vi "Engine-RPC-SyncPumpA.vi"(8 "Error In":errorcluster, 11 "DSI Reference":refnum<class "DCM-DSI.lvclass">) -> (0 "Error Out":errorcluster, 3 "DSI Reference":refnum<class "DCM-DSI.lvclass">)   [LabVIEW 2016, in "DSI-RT.lvlib"]
uses:
  DSI-RT.lvlib
  Classes/DCM-DSI/DCM-DSI.lvclass
  <vilib>/addons/Software Calibration Management/xSCM/Controls/TBL2D.ctl
  <vilib>/Powertrain Controls/Device Drivers/DCM/Rev0/RT/DCM - RT.lvclass/DCM - RT.ctl
  <vilib>/Powertrain Controls/Device Drivers/DCM/Rev0/RT/Read Max CAD.vi
  Classes/DCM-DSI/Read DiffIO Results.vi
  Classes/DCM-DSI/Read DCM Ref.vi
  Classes/DCM-DSI/Read EPTx Data.vi
  Classes/DCM-DSI/Read Channels.vi
  Classes/DCM-DSI/Read dt.vi
  Classes/DCM-DSI/Write Pump-A Command.vi
  <vilib>/Powertrain Controls/Device Drivers/DCM/Rev0/RT/DCM - RT.lvclass
  <vilib>/addons/Software Calibration Management/xSCM/FaultPoint.xnode
  <vilib>/addons/Software Calibration Management/xSCM/CalPoint.xnode
  <vilib>/addons/Software Calibration Management/xSCM/Controls/TLU2D.ctl
  <vilib>/addons/Software Calibration Management/xSCM/ni_scm.dll
  <vilib>/addons/Software Calibration Management/xSCM/SCM-API.lvlib
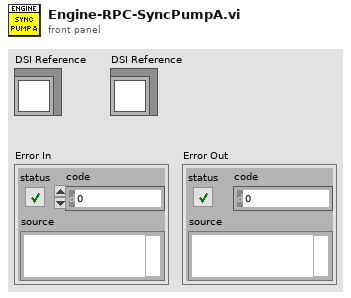
[diagram p1: front panel]
types:
  T1 = cluster{"PID_Kp":sgl, "PID_Ti":sgl, "PID_Td":sgl, "PID_FF":sgl, "Non-PID_FF":sgl, "PID_Min":sgl, "PID_Max":sgl}
  T2 = typedef "DCM - RT - Diff IO.lvlib/Results.ctl" = cluster{"Capture [DBTDC]":sgl, "Capture Error":bool, "Frequency [Hz]":sgl, "Duty Cycle [%]":sgl, "PWM Stopped":bool}
  T3 = typedef "EPTx - RevA - RT.lvlib/EPTxData.ctl" = cluster{"Sync":bool, "CurrentCAD":sgl, "Speed [RPM]":sgl, "Config":bool, "Rcvg Primary":bool, "Stall":bool, "Overflow":bool, "Ratio Error":bool, "Pattern Error":bool, "Aux Warning":bool, "Watchdog Error":bool}
  T4 = typedef "DCM-DSI.lvclass/Channel.ctl" = cluster{"Name":string, "Unit":string, "Value":sgl}
  T5 = typedef "DSI-Shared.lvlib/Engine-Channel.ctl" = cluster{"Name":string, "Unit":string, "Value":sgl}
  T6 = typedef "SCM-API.lvlib/TBL2D.ctl" = cluster{"X":sgl[], "Y":sgl[], "Z":sgl[][]}
  T7 = typedef "SCM-API.lvlib/TLU2D.ctl" = cluster{"X":sgl, "Y":sgl, "Z":sgl}
  T8 = cluster{"Duration":cluster{"Dur_Max":sgl, "Dur_Min":sgl, "Dur_ManE":bool, "Dur_Man":sgl}, "Timing":cluster{"WindowStart":sgl, "WindowEnd":sgl, "EndAngle?":bool, "DurAngle_Max":sgl, "MinOffTime":sgl}}
  T9 = cluster{"Dur_Max":sgl, "Dur_Min":sgl, "Dur_ManE":bool, "Dur_Man":sgl}
  T10 = cluster{"WindowStart":sgl, "WindowEnd":sgl, "EndAngle?":bool, "DurAngle_Max":sgl, "MinOffTime":sgl}
  T11 = cluster{"ProportionalAction":sgl, "IntegralAction":sgl, "DerivativeAction":sgl}
  T12 = enum8{"Unused", "User OS", "Diff IO 1", "Diff IO 2", "Diff IO 3", "Diff IO 4", "Diff IO 5", "Diff IO 6", "Diff IO 7", "Diff IO 8", "Aux 1", "Aux 2", "Aux 3", "Aux 4", "Aux 5", "Aux 6", "Aux 7", "Aux 8", "Aux 9", "Aux 10", "Aux 11", "Aux 12", "Aux 13", "Aux 14", "Aux 15", "Aux 16"}
  T13 = cluster{"Value":enum8{"Unused", "User OS", "Diff IO 1", "Diff IO 2", "Diff IO 3", "Diff IO 4", "Diff IO 5", "Diff IO 6", "Diff IO 7", "Diff IO 8", "Aux 1", "Aux 2", "Aux 3", "Aux 4", "Aux 5", "Aux 6", "Aux 7", "Aux 8", "Aux 9", "Aux 10", "Aux 11", "Aux 12", "Aux 13", "Aux 14", "Aux 15", "Aux 16"}, "Value":sgl}
  T14 = cluster{"Value":sgl, "Value":sgl, "Duration_Output":sgl}
  T15 = typedef "DCM - RT - DI.lvlib/Command.ctl" = cluster{"Mode":T16, "Digital Input":T17, "Default Profile Index":u8, "Cal Freq [Hz]":sgl, "Cal Duration [s]":sgl, "Cal Increment [s]":sgl, "Cal Pulses":u16, "TMP Command Sequence":T18[], "EPT TDC Offset [CAD]":sgl, "EPT Window Start [DBTDC]":sgl, "EPT Window End [DBTDC]":sgl, "EPT Angles":T19[], "EPT Skip Fire":bool, "EPT Skip Index":u8, "EPT Precharge Duration [s]":sgl, "EPT Precharge Profile Index":u8}
  T16 = typedef "DCM - FPGA - DI.lvlib/Mode.ctl" = enum8{"Off", "Direct", "Calibration", "Triggered Multi-Pulse", "Engine Position Tracking"}
  T17 = typedef "DCM - FPGA.lvlib/Digital Channel.ctl" = enum8{"Unused", "User OS", "Diff IO 1", "Diff IO 2", "Diff IO 3", "Diff IO 4", "Diff IO 5", "Diff IO 6", "Diff IO 7", "Diff IO 8", "Aux 1", "Aux 2", "Aux 3", "Aux 4", "Aux 5", "Aux 6", "Aux 7", "Aux 8", "Aux 9", "Aux 10", "Aux 11", "Aux 12", "Aux 13", "Aux 14", "Aux 15", "Aux 16"}
  T18 = typedef "DCM - RT - DI.lvlib/Command Sequence.ctl" = cluster{"Duration [s]":sgl, "Level":bool, "Run/Stop":bool, "Profile Index":u8}
  T19 = typedef "DCM - RT - DI.lvlib/Angle Control.ctl" = cluster{"Enable":bool, "Timing [DBTDC]":sgl, "Duration [s]":sgl, "Profile Index":u8}
  T20 = cluster{"Sync-A_Timing":sgl, "Sync-A_CamAdv":sgl}
  T21 = cluster{"Output":cluster{"Duration_Output":sgl, "PID_Output":sgl}, "EPT Mode Output":cluster{"Sync-A_Timing":sgl, "Sync-A_CamAdv":sgl}, "TMP Mode Output":cluster{"Sync-A_Delay":sgl, "Sync-A_Period":sgl}}
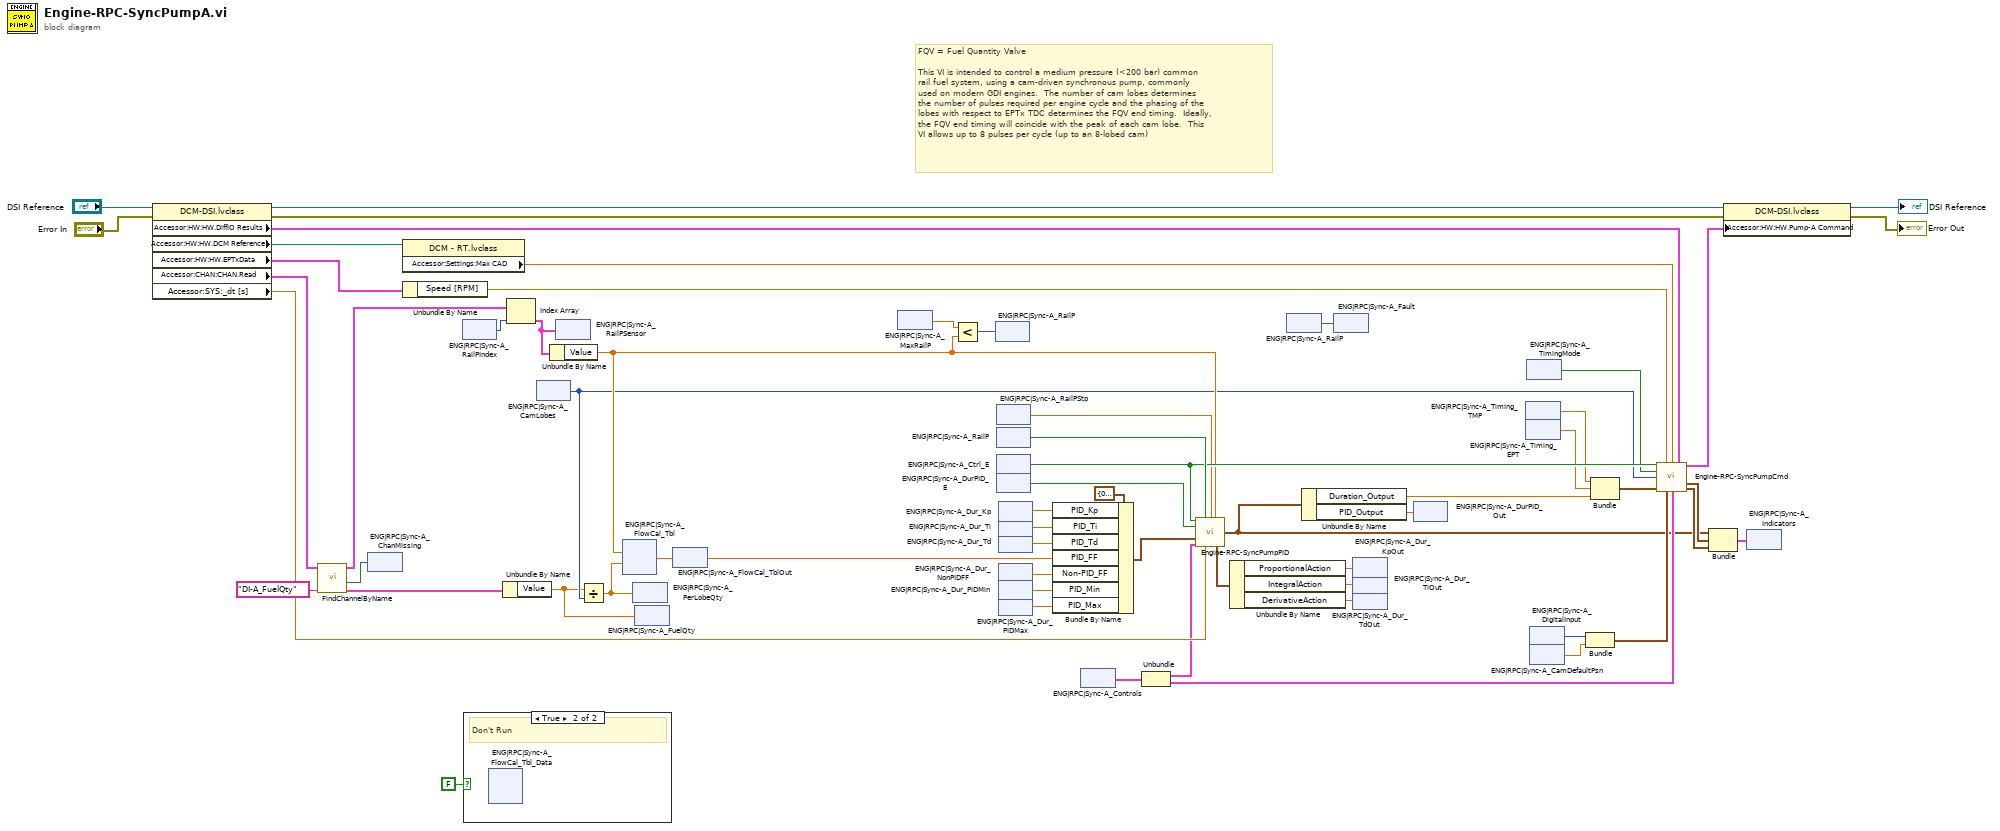
[diagram p0: block diagram]
diagram:
  # "FQV = Fuel Quantity Valve\n\nThis VI is intended to control a medium pressure (<200 bar) common\nrail fuel system, using a cam-driven synchronous pump, commonly\nused on modern GDI engines.  The number of cam lobes determines \nthe number of pulses required per engine cycle and the phasing of the\nlobes with respect to EPTx TDC determines the FQV end timing.  Ideally,\nthe FQV end timing will coincide with the peak of each cam lobe.  This\nVI allows up to 8 pulses per cycle (up to an 8-lobed cam)"
  n1 = property class="DCM-DSI.lvclass"(reference="DSI Reference", error in="Error In") -> (reference out=w44:refnum<class "DCM-DSI.lvclass">, error out=w43:errorcluster, "Accessor:HW:HW.DiffIO Results"=w30:T2[], "Accessor:HW:HW.DCM Reference"=w31:refnum<class "DCM - RT.lvclass">, "Accessor:HW:HW.EPTxData"=w42:T3, "Accessor:CHAN:CHAN.Read"=w7:T4[], "Accessor:SYS:_dt [s]"=w39:sgl)
  n2 = call "FindChannelByName.vi"("Name"="DI-A_FuelQty", "CTRL.Channels in"=w7) -> ("Channel"=w9:T5, "Searching"=w5:bool, "CTRL.Channels out"=w4:T5[])  [unwired: 6 in, 1 out]
  n3 = xnode "ENG|RPC|Sync-A_ChanMissing"("Fault"=w5) -> ()
  n4 = property class="DCM - RT.lvclass"(reference=w31) -> ("Accessor:Settings:Max CAD"=w32:sgl)  [unwired: 1 in, 2 out]
  n5 = Unbundle By Name(w42) -> ("Speed [RPM]"=w35:sgl)
  n6 = xnode "ENG|RPC|Sync-A_RailPIndex"() -> ("Value"=w3:i32)
  n7 = case shown="True" FALSE {
    frame False {
    }
    frame True {
      # "Don't Run"
      n8 = xnode "ENG|RPC|Sync-A_FlowCal_Tbl_Data"() -> ()  [unwired: 1 out]
    }
  }
  n9 = Unbundle By Name(w9) -> ("Value"=w10:sgl)
  n10 = Index Array(array=w4, index=w3) -> (element=w2:T5)
  n11 = xnode "ENG|RPC|Sync-A_CamLobes"() -> ("Value"=w20:u8)
  n12 = Unbundle By Name(w2) -> ("Value"=w21:sgl)
  n13 = xnode "ENG|RPC|Sync-A_RailPSensor"("Value"=w2) -> ()
  n14 = Divide(x=w10, y=w20) -> (x/y=w37:sgl)
  n15 = xnode "ENG|RPC|Sync-A_FlowCal_Tbl"("Y Index"=w37, "X Index"=w21) -> ("Z"=w45:sgl)
  n16 = xnode "ENG|RPC|Sync-A_PerLobeQty"("Value"=w37) -> ()
  n17 = xnode "ENG|RPC|Sync-A_FuelQty"("Value"=w10) -> ()
  n18 = xnode "ENG|RPC|Sync-A_FlowCal_TblOut"("Value"=w45) -> ()
  n19 = xnode "ENG|RPC|Sync-A_MaxRailP"() -> ("Value"=w22:sgl)
  n20 = Less?(x=w22, y=w21) -> (x < y?=w41:bool)
  n21 = xnode "ENG|RPC|Sync-A_RailP"("Fault"=w41) -> ()
  n22 = xnode "ENG|RPC|Sync-A_RailPStp"() -> ("Value"=w12:sgl)
  n23 = xnode "ENG|RPC|Sync-A_RailP"() -> ("Fault"=w40:bool)
  n24 = xnode "ENG|RPC|Sync-A_Ctrl_E"() -> ("Value"=w36:bool)
  n25 = xnode "ENG|RPC|Sync-A_DurPID_E"() -> ("Value"=w46:bool)
  n26 = xnode "ENG|RPC|Sync-A_Dur_Kp"() -> ("Value"=w50:sgl)
  n27 = xnode "ENG|RPC|Sync-A_Dur_Ti"() -> ("Value"=w51:sgl)
  n28 = xnode "ENG|RPC|Sync-A_Dur_Td"() -> ("Value"=w52:sgl)
  n29 = xnode "ENG|RPC|Sync-A_Dur_NonPIDFF"() -> ("Value"=w38:sgl)
  n30 = xnode "ENG|RPC|Sync-A_Dur_PIDMin"() -> ("Value"=w53:sgl)
  n31 = xnode "ENG|RPC|Sync-A_Dur_PIDMax"() -> ("Value"=w54:sgl)
  n32 = Bundle By Name(cluster=T1 {"PID_Kp"=0.0, "PID_Ti"=0.01, "PID_Td"=0.0, "PID_FF"=0.0, "Non-PID_FF"=0.0, "PID_Min"=-100.0, "PID_Max"=100.0} ("PID Settings"), "PID_Kp"=w50, "PID_Ti"=w51, "PID_Td"=w52, "PID_FF"=w45, "Non-PID_FF"=w38, "PID_Min"=w53, "PID_Max"=w54) -> (w47:T1)
  n33 = xnode "ENG|RPC|Sync-A_Controls"() -> ("Value"=w19:T8)
  n34 = Unbundle(w19) -> ("Duration"=w18:T9, "Timing"=w17:T10)
  n35 = call "Engine-RPC-SyncPumpPID.vi"("Control Enable"=w36, "Fault Input"=w40, "Rail Press Setpoint"=w12, "Rail Pressure"=w21, "PID Enable"=w46, "PID Settings"=w47, "Output Management Controls"=w18, "dt (s)"=w39) -> ("Output"=w14:cluster{"Duration_Output":sgl, "PID_Output":sgl}, "PID_Action_Output"=w49:T11)  [unwired: 6 in]
  n36 = Unbundle By Name(w49) -> ("ProportionalAction"=w57:sgl, "IntegralAction"=w56:sgl, "DerivativeAction"=w55:sgl)
  n37 = xnode "ENG|RPC|Sync-A_RailP"() -> ("Fault"=w6:bool)
  n38 = Unbundle By Name(w14) -> ("Duration_Output"=w24:sgl, "PID_Output"=w11:sgl)
  n39 = xnode "ENG|RPC|Sync-A_Fault"("Value"=w6) -> ()
  n40 = xnode "ENG|RPC|Sync-A_Dur_KpOut"("Value"=w57) -> ()
  n41 = xnode "ENG|RPC|Sync-A_Dur_TiOut"("Value"=w56) -> ()
  n42 = xnode "ENG|RPC|Sync-A_Dur_TdOut"("Value"=w55) -> ()
  n43 = xnode "ENG|RPC|Sync-A_DurPID_Out"("Value"=w11) -> ()
  n44 = xnode "ENG|RPC|Sync-A_Timing_TMP"() -> ("Value"=w26:sgl)
  n45 = xnode "ENG|RPC|Sync-A_Timing_EPT"() -> ("Value"=w25:sgl)
  n46 = xnode "ENG|RPC|Sync-A_TimingMode"() -> ("Value"=w27:bool)
  n47 = xnode "ENG|RPC|Sync-A_DigitalInput"() -> ("Value"=w34:T12)
  n48 = xnode "ENG|RPC|Sync-A_CamDefaultPsn"() -> ("Value"=w33:sgl)
  n49 = Bundle("Value"=w34, "Value"=w33) -> (w28:T13)  [unwired: 1 in]
  n50 = Bundle("Value"=w26, "Value"=w25, "Duration_Output"=w24) -> (w23:T14)  [unwired: 1 in]
  n51 = call "Engine-RPC-SyncPumpCmd.vi"("FQV Enable"=w36, "Engine Speed [RPM]"=w35, "MaxCAD"=w32, "HW.DiffIO Results"=w30, "Mode [T=Trig,F=EPT]"=w27, "Cam Lobes"=w20, "Command"=w23, "DigitalInputSettings"=w28, "EPT Mode Settings"=w17) -> ("Pump Command"=w29:T15, "EPT Mode Output"=w16:T20, "TMP Mode Output"=w15:cluster{"Sync-A_Delay":sgl, "Sync-A_Period":sgl})  [unwired: 4 in]
  n52 = Bundle("Output"=w14, "EPT Mode Output"=w16, "TMP Mode Output"=w15) -> (w13:T21)  [unwired: 1 in]
  n53 = property class="DCM-DSI.lvclass"(reference=w44, error in=w43, "Accessor:HW:HW.Pump-A Command"=w29) -> (reference out=→"DSI Reference":refnum<class "DCM-DSI.lvclass">, error out=→"Error Out":errorcluster)
  n54 = xnode "ENG|RPC|Sync-A_Indicators"("Value"=w13) -> ()
